vi "浏览器.vi"() -> ()   [LabVIEW 2018]
panel:
  in  "刷新按钮":bool
  in  "停止按钮":bool
  in  "向下按钮":bool
  in  "网址：":string
  in  "WebBrowser":refnum<k7>(container) caption="网页浏览器"
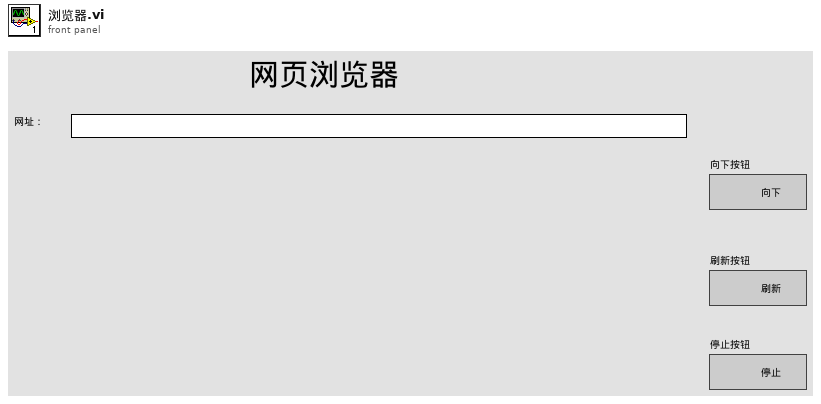
[diagram p1: front panel]
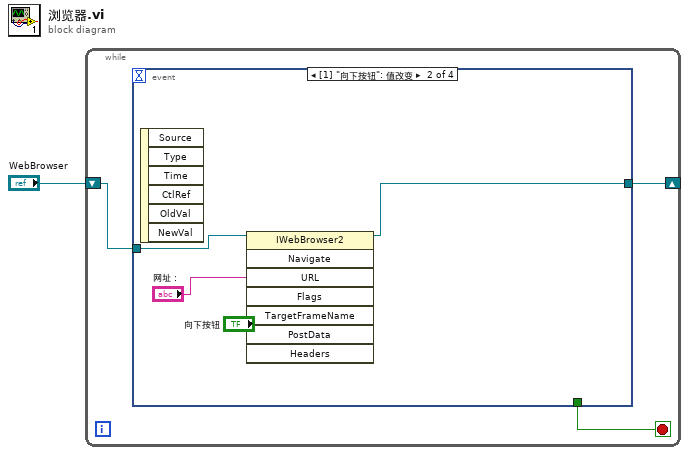
[diagram p0: block diagram]
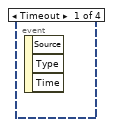
[diagram p2: hidden frame]
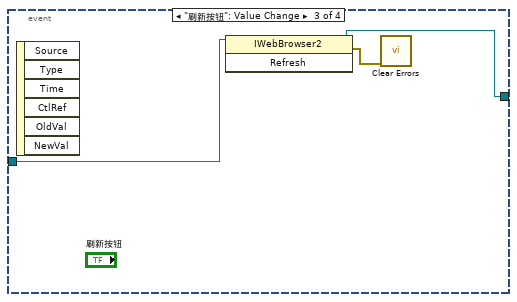
[diagram p3: hidden frame]
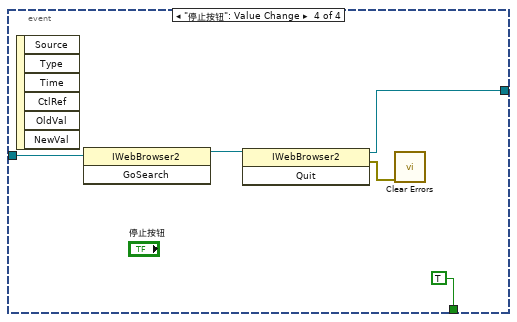
[diagram p4: hidden frame]
diagram:
  n1 = while {
    shift-right: [w3] -> _
    shift-left: "WebBrowser" -> [w4]
    stop <- w2 stop-if-true
    n2 = event shown="[1] \"向下按钮\": 值改变" {
      selector: _ -> [_ _ _ _]
      dyn-events: _ -> [_ _ _ _]
      timeout: _ -> [_ _ _ _]
      tunnel: w4 -> [_ w7 w10 w15]
      tunnel: [_ w6 w9 w13] -> w3
      tunnel: [_ _ _ TRUE] -> w2
      event Timeout {
        n3 = event-data() -> ()  [unwired: 1 in, 3 out]
      }
      event "向下按钮": Value Change {
        n4 = event-data() -> ()  [unwired: 1 in, 6 out]
        n5 = invoke class="IWebBrowser2" method="Navigate"(reference=w7, "URL"="网址：") -> (reference out=w6:refnum<k7>)  [unwired: 6 in, 7 out]
      }
      event "刷新按钮": Value Change {
        n6 = event-data() -> ()  [unwired: 1 in, 6 out]
        n7 = invoke class="IWebBrowser2" method="Refresh"(reference=w10) -> (reference out=w9:refnum<k7>, error out=w8:errorcluster)  [unwired: 2 in, 1 out]
        n8 = call <vilib>:"Clear Errors.vi"("error in (no error)"=w8) -> ()  [unwired: 5 in, 2 out]
      }
      event "停止按钮": Value Change {
        n9 = event-data() -> ()  [unwired: 1 in, 6 out]
        n10 = invoke class="IWebBrowser2" method="GoSearch"(reference=w15) -> (reference out=w14:refnum<k7>)  [unwired: 2 in, 2 out]
        n11 = invoke class="IWebBrowser2" method="Quit"(reference=w14) -> (reference out=w13:refnum<k7>, error out=w12:errorcluster)  [unwired: 2 in, 1 out]
        n12 = call <vilib>:"Clear Errors.vi"("error in (no error)"=w12) -> ()  [unwired: 5 in, 2 out]
      }
    }
  }
